vi "Read Exporter Path.vi"(11 "CDependencyInspection in":refnum<class "CDependencyInspection.lvclass">) -> (2 "Path":path, 3 "CDependencyInspection out":refnum<class "CDependencyInspection.lvclass">)   [LabVIEW 2020, in "DependencyInspection.lvlib" / "CDependencyInspection.lvclass"]
uses:
  CDependencyInspection.lvclass
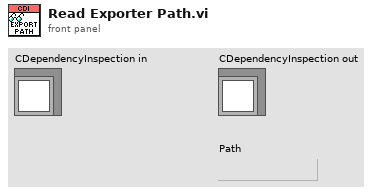
[diagram p1: front panel]
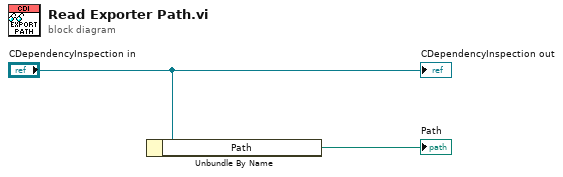
[diagram p0: block diagram]
diagram:
  n1 = Unbundle By Name("CDependencyInspection in") -> ("Path"=→"Path":path)
  "CDependencyInspection out" <- "CDependencyInspection in"
